vi "wind turbine performance simulation.vi"() -> ()   [LabVIEW 2018]
uses:
  <vilib>/Utility/file.llb/Read Delimited Spreadsheet (DBL).vi
panel:
  out "Numeric 2":dbl
  out "Actual Power (KW)":dbl(knob) scale=0.0..1.0
  out "Numeric":dbl
  out "Power Generated (KW)":dbl(graph)
  out "Data Table":dbl[][](array[numeric])
  out "Speed Guage -\nBlades Failure for Speeds Above 10":dbl(knob) scale=0.0..24.0
  out "Power Generated (KW)":dbl(knob) scale=0.0..1.5
  out "Speed":dbl(graph)
  out "Blades":bool
  out "Ring":u16(ring)
  in  "Wind Speed        Time (hr)":dbl[](array[slide]) scale=0.0..14.0
  out "Turbine Height for Optimal Power generation":i32[](array[numeric])
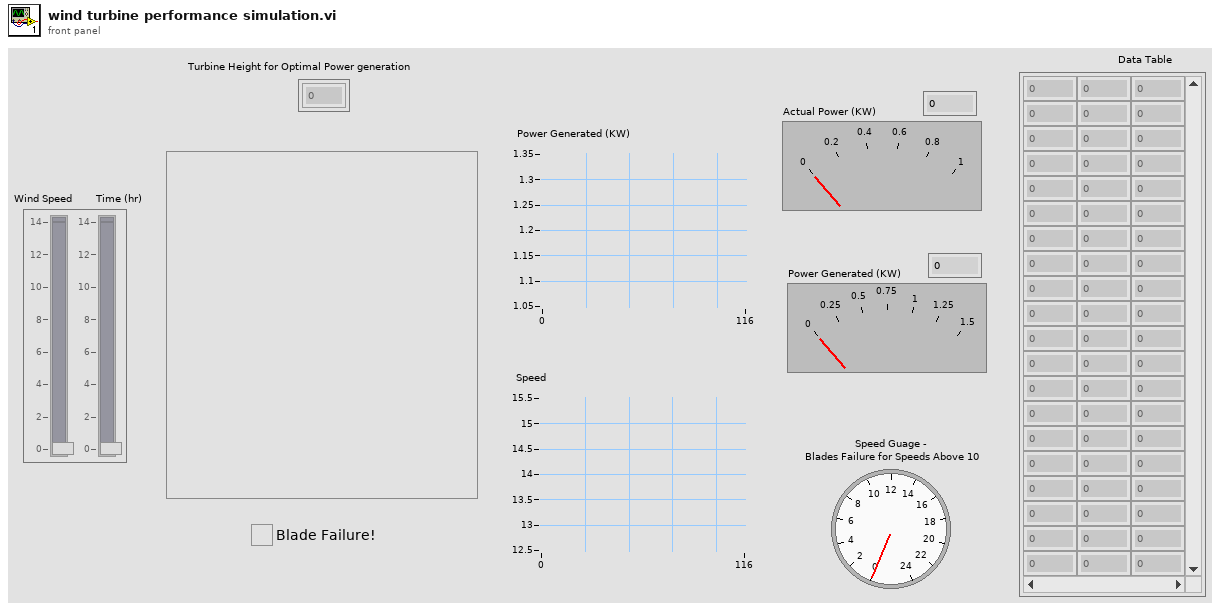
[diagram p1: front panel]
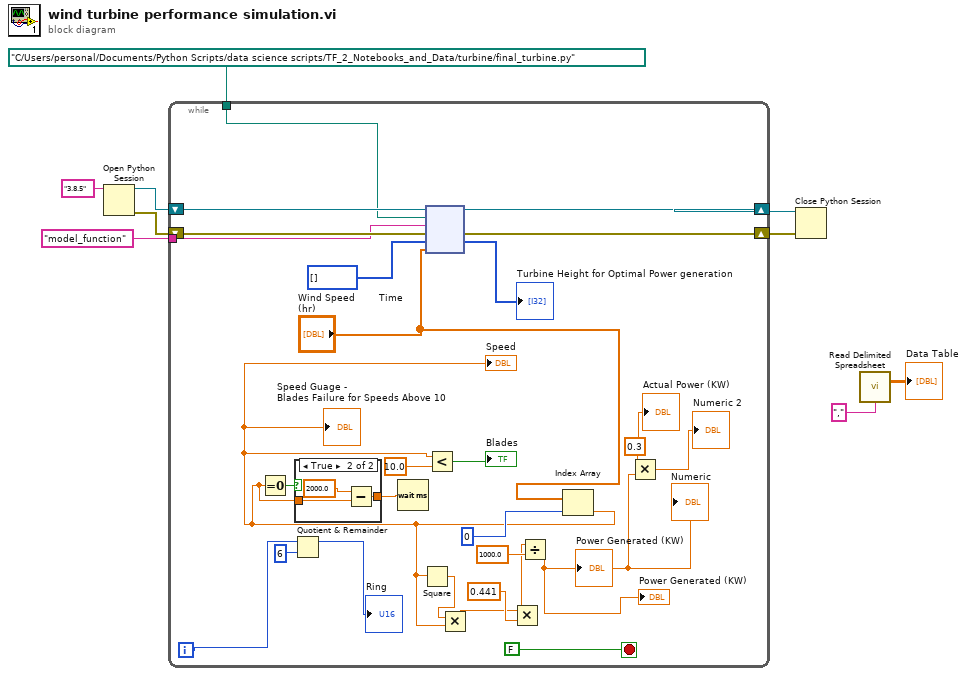
[diagram p0: block diagram]
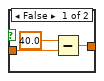
[diagram p2: hidden frame]
diagram:
  n1 = Open Python Session(python version="3.8.5" ("Python version")) -> (session out=w9:refnum<k35>, error out=w8:errorcluster)  [unwired: 2 in]
  n2 = while {
    tunnel: path "C:/Users/personal/Documents/Python Scripts/data science scripts/TF_2_Notebooks_and_Data/turbine/final_turbine.py" ("module path") -> [w32]
    tunnel: "model_function" ("function name") -> [w31]
    shift-right: [w34] -> w7
    shift-left: w9 -> [w36]
    shift-right: [w33] -> w6
    shift-left: w8 -> [w35]
    i -> [w23]
    stop <- FALSE stop-if-true
    n3 = Quotient & Remainder(x=w23, y=6) -> (x-y*floor(x/y)=→"Ring":i32)  [unwired: 1 out]
    n4 = node(w36, w32, w31, w35, i32[] [], "Wind Speed        Time (hr)") -> (w34:refnum<k35>, w33:errorcluster, →"Turbine Height for Optimal Power generation":i32[])  [unwired: 1 in, 2 out]
    n5 = Index Array(array="Wind Speed        Time (hr)", index=0) -> (element=w13:dbl)
    "Speed" <- w13
    "Speed Guage -\nBlades Failure for Speeds Above 10" <- w13
    n6 = Equal To 0?(x=w13) -> (x = 0?=w18:bool)
    n7 = case shown="True" w18 {
      tunnel: [w39 w41] -> w19
      tunnel: w13 -> [w37 w40]
      frame False {
        n8 = Subtract(x=40.0, y=w37) -> (x-y=w39:dbl)
      }
      frame True {
        n9 = Subtract(x=2000.0, y=w40) -> (x-y=w41:dbl)
      }
    }
    n10 = Wait (ms)(milliseconds to wait=w19) -> ()  [unwired: 1 out]
    n11 = Square(x=w13) -> (x^2=w15:dbl)
    n12 = Less?(x=w13, y=10.0) -> (x < y?=→"Blades":bool)
    n13 = Multiply(x=w15, y=w13) -> (x*y=w14:dbl)
    n14 = Multiply(x=w14, y=0.441) -> (x*y=w16:dbl)
    n15 = Divide(x=w16, y=1000.0) -> (x/y=w12:dbl)
    "Power Generated (KW)" <- w12
    "Power Generated (KW)" <- w12
    "Numeric" <- w12
    n16 = Multiply(x=0.3, y=w12) -> (x*y=→"Actual Power (KW)" →"Numeric 2":dbl)
  }
  n17 = Close Python Session(session in=w7, error in=w6) -> ()  [unwired: 1 out]
  n18 = call-poly <vilib>:"Read Delimited Spreadsheet.vi"("delimiter (\\t)"="," ("delimiter (\\t)")) -> ("all rows"=→"Data Table":dbl[][])  [unwired: 9 in, 5 out]
